vi "Nr_of_next_Motor_Scan.vi"(7 "Scan Type":u16(ring) items=["Energy / Time", "Motor", "TDC", "Keithley"], 8 "error in (no error)":errorcluster, 11 "base path":path=path "C:/Users/ALS Measurement/Google Drive/DATA") -> (0 "error out":errorcluster, 2 "scan nr":i32, 3 "path out":path)   [LabVIEW 2018]
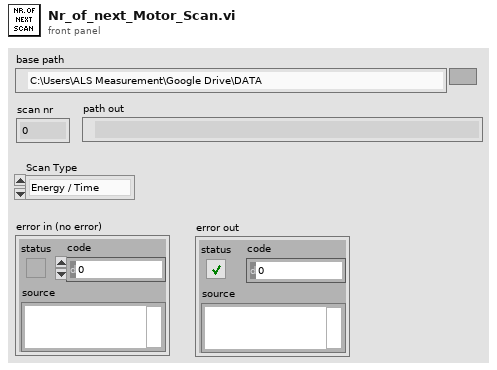
[diagram p1: front panel]
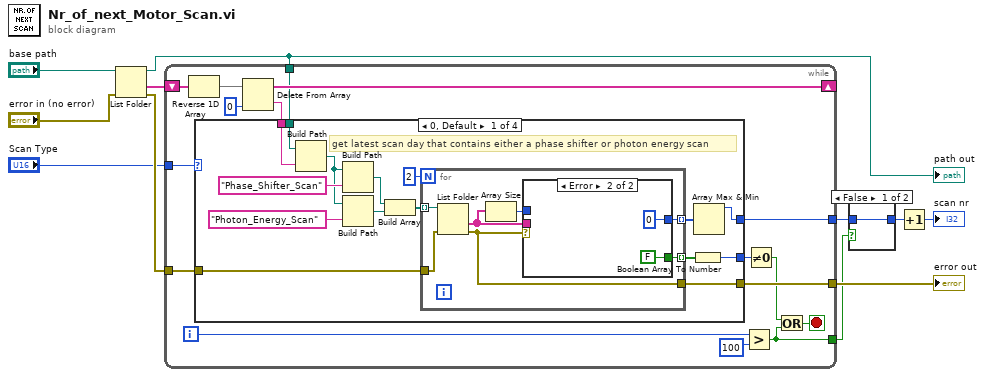
[diagram p0: block diagram]
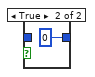
[diagram p2: hidden frame]
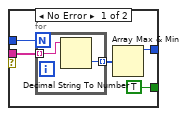
[diagram p3: hidden frame]
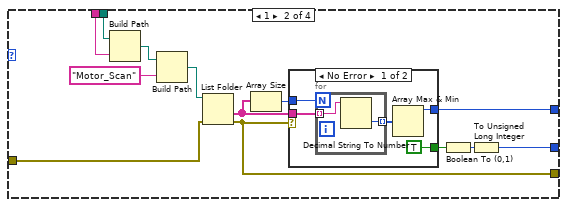
[diagram p4: hidden frame]
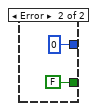
[diagram p5: hidden frame]
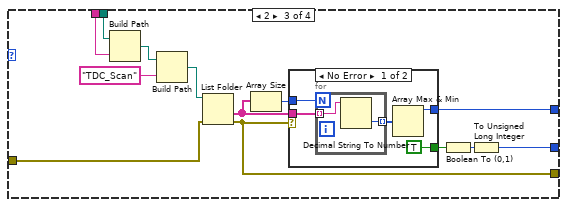
[diagram p6: hidden frame]
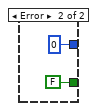
[diagram p7: hidden frame]
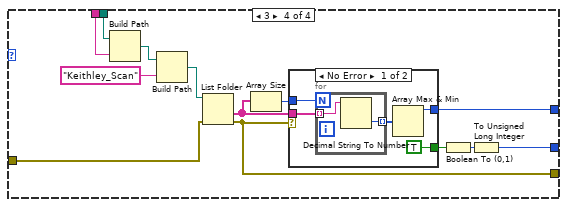
[diagram p8: hidden frame]
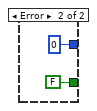
[diagram p9: hidden frame]
diagram:
  n1 = List Folder(path="base path", error in="error in (no error)") -> (path out=w7:path, folder names=w10:string[], error out=w9:errorcluster)  [unwired: 2 in, 1 out]
  "path out" <- w7
  n2 = while {
    shift-right: [w24] -> _
    shift-left: w10 -> [w27]
    tunnel: w9 -> [w23]
    tunnel: [w15] -> w1
    tunnel: [w17] -> w5
    tunnel: w7 -> [w19]
    tunnel: "Scan Type" -> [w13]
    tunnel: [w12] -> w3
    i -> [w22]
    stop <- w20 stop-if-true
    n3 = Reverse 1D Array(array=w27) -> (reversed array=w26:string[])
    n4 = Delete From Array(array=w26, index=0) -> (deleted portion=w18:string, array with subset deleted=w24:string[])  [unwired: 1 in]
    n5 = case shown="0, Default" w13 {
      tunnel: w23 -> [w37 w70 w92 w114]
      tunnel: w19 -> [w36 w69 w91 w113]
      tunnel: w18 -> [w35 w68 w90 w112]
      tunnel: [w33 w66 w88 w110] -> w17
      tunnel: [w30 w60 w82 w104] -> w16
      tunnel: [w28 w64 w86 w108] -> w15
      frame 0, Default {
        # "get latest scan day that contains either a phase shifter or photon energy scan"
        n6 = Build Path(base path=w36, name or relative path=w35) -> (appended path=w34:path)
        n7 = Build Path(base path=w34, name or relative path="Phase_Shifter_Scan") -> (appended path=w40:path)
        n8 = Build Path(base path=w34, name or relative path="Photon_Energy_Scan") -> (appended path=w39:path)
        n9 = Build Array(w40, w39) -> (w38:path[])
        n10 = for {
          N: 2 -> [_]
          tunnel: w38 -> [w47] mode=indexing
          tunnel: [w49] -> w29 mode=indexing
          tunnel: w37 -> [w48]
          tunnel: [w44] -> w33
          tunnel: [w43] -> w31 mode=indexing
          n11 = List Folder(path=w47, error in=w48) -> (folder names=w46:string[], error out=w44:errorcluster)  [unwired: 2 in, 2 out]
          n12 = Array Size(array=w46) -> (size(s)=w45:i32)
          n13 = case shown="Error" w44 {
            tunnel: [w54 0] -> w49
            tunnel: w46 -> [w52 _]
            tunnel: w45 -> [w51 _]
            tunnel: [TRUE FALSE] -> w43
            frame No Error {
              n14 = for {
                N: w51 -> [_]
                tunnel: w52 -> [w56] mode=indexing
                tunnel: [w55] -> w53 mode=indexing
                n15 = Decimal String To Number(string=w56) -> (number=w55:i32)  [unwired: 2 in, 1 out]
              }
              n16 = Array Max & Min(array=w53) -> (max value=w54:i32)  [unwired: 3 out]
            }
            frame Error {
            }
          }
        }
        n17 = Boolean Array To Number(Boolean array=w31) -> (number=w30:u32)
        n18 = Array Max & Min(array=w29) -> (max value=w28:i32)  [unwired: 3 out]
      }
      frame 1 {
        n19 = Build Path(base path=w69, name or relative path=w68) -> (appended path=w67:path)
        n20 = Build Path(base path=w67, name or relative path="Motor_Scan") -> (appended path=w59:path)
        n21 = List Folder(path=w59, error in=w70) -> (folder names=w63:string[], error out=w66:errorcluster)  [unwired: 2 in, 2 out]
        n22 = Array Size(array=w63) -> (size(s)=w62:i32)
        n23 = case shown="No Error" w66 {
          tunnel: [w76 0] -> w64
          tunnel: w63 -> [w74 _]
          tunnel: w62 -> [w73 _]
          tunnel: [TRUE FALSE] -> w65
          frame No Error {
            n24 = for {
              N: w73 -> [_]
              tunnel: w74 -> [w78] mode=indexing
              tunnel: [w77] -> w75 mode=indexing
              n25 = Decimal String To Number(string=w78) -> (number=w77:i32)  [unwired: 2 in, 1 out]
            }
            n26 = Array Max & Min(array=w75) -> (max value=w76:i32)  [unwired: 3 out]
          }
          frame Error {
          }
        }
        n27 = Boolean To (0,1)(Boolean=w65) -> (0, 1=w61:i16)
        n28 = To Unsigned Long Integer(number=w61) -> (unsigned 32bit integer=w60:u32)
      }
      frame 2 {
        n29 = Build Path(base path=w91, name or relative path=w90) -> (appended path=w89:path)
        n30 = Build Path(base path=w89, name or relative path="TDC_Scan") -> (appended path=w81:path)
        n31 = List Folder(path=w81, error in=w92) -> (folder names=w85:string[], error out=w88:errorcluster)  [unwired: 2 in, 2 out]
        n32 = Array Size(array=w85) -> (size(s)=w84:i32)
        n33 = case shown="No Error" w88 {
          tunnel: [w98 0] -> w86
          tunnel: w85 -> [w96 _]
          tunnel: w84 -> [w95 _]
          tunnel: [TRUE FALSE] -> w87
          frame No Error {
            n34 = for {
              N: w95 -> [_]
              tunnel: w96 -> [w100] mode=indexing
              tunnel: [w99] -> w97 mode=indexing
              n35 = Decimal String To Number(string=w100) -> (number=w99:i32)  [unwired: 2 in, 1 out]
            }
            n36 = Array Max & Min(array=w97) -> (max value=w98:i32)  [unwired: 3 out]
          }
          frame Error {
          }
        }
        n37 = Boolean To (0,1)(Boolean=w87) -> (0, 1=w83:i16)
        n38 = To Unsigned Long Integer(number=w83) -> (unsigned 32bit integer=w82:u32)
      }
      frame 3 {
        n39 = Build Path(base path=w113, name or relative path=w112) -> (appended path=w111:path)
        n40 = Build Path(base path=w111, name or relative path="Keithley_Scan") -> (appended path=w103:path)
        n41 = List Folder(path=w103, error in=w114) -> (folder names=w107:string[], error out=w110:errorcluster)  [unwired: 2 in, 2 out]
        n42 = Array Size(array=w107) -> (size(s)=w106:i32)
        n43 = case shown="No Error" w110 {
          tunnel: [w120 0] -> w108
          tunnel: w107 -> [w118 _]
          tunnel: w106 -> [w117 _]
          tunnel: [TRUE FALSE] -> w109
          frame No Error {
            n44 = for {
              N: w117 -> [_]
              tunnel: w118 -> [w122] mode=indexing
              tunnel: [w121] -> w119 mode=indexing
              n45 = Decimal String To Number(string=w122) -> (number=w121:i32)  [unwired: 2 in, 1 out]
            }
            n46 = Array Max & Min(array=w119) -> (max value=w120:i32)  [unwired: 3 out]
          }
          frame Error {
          }
        }
        n47 = Boolean To (0,1)(Boolean=w109) -> (0, 1=w105:i16)
        n48 = To Unsigned Long Integer(number=w105) -> (unsigned 32bit integer=w104:u32)
      }
    }
    n49 = Greater?(x=w22, y=100) -> (0:w12:bool)
    n50 = Not Equal To 0?(x=w16) -> (x != 0?=w14:bool)
    n51 = Or(x=w14, y=w12) -> (x .or. y?=w20:bool)
  }
  "error out" <- w5
  n52 = case shown="False" w3 {
    tunnel: [w125 0 ("x")] -> w2
    tunnel: w1 -> [w125 _]
    frame False {
    }
    frame True {
    }
  }
  n53 = Increment(x=w2) -> (x+1=→"scan nr":i32)
